vi "Vector2DMagnitude.vi"(10 "Vector":T1) -> (2 "Magnitude":dbl)   [LabVIEW 2018]
uses:
  Vector2D.ctl
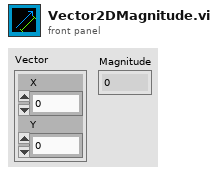
[diagram p1: front panel]
types:
  T1 = typedef "Vector2D.ctl" = cluster{"X":dbl, "Y":dbl}
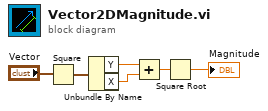
[diagram p0: block diagram]
diagram:
  n1 = Square(x="Vector") -> (x^2=w4:T1)
  n2 = Unbundle By Name(w4) -> ("Y"=w2:dbl, "X"=w1:dbl)
  n3 = Add(x=w2, y=w1) -> (x+y=w5:dbl)
  n4 = Square Root(x=w5) -> (sqrt(x)=→"Magnitude":dbl)
